vi "Out_S2F23.vi"(8 "error in (no error)":errorcluster, 10 "S2F23":T1, 11 "S2 Message Class in":refnum<class "S2 Message Class.lvclass">) -> (0 "error out":errorcluster, 3 "S2 Message Class out":refnum<class "S2 Message Class.lvclass">)   [LabVIEW 2020, in "SECS Communication.lvlib" / "S2 Message Class.lvclass"]
uses:
  S2 Message Class.lvclass
  D:/Dropbox/SECS/SECS_GEM v1.0.6/Com/SECS Communication/SECS-II Class/SECS-II Class.lvclass
  S2F23.ctl
  SECS-II Class/Data Message_List.vi
  SECS-II Class/Data Message_U4.vi
  SECS-II Class/Data Message_ASCII.vi
  SECS-II Class/SECS-II Class.lvclass
  D:/Dropbox/SECS/SECS_GEM v1.0.6/Com/SECS Communication/S2 Message Class/S2 Message Class.lvclass
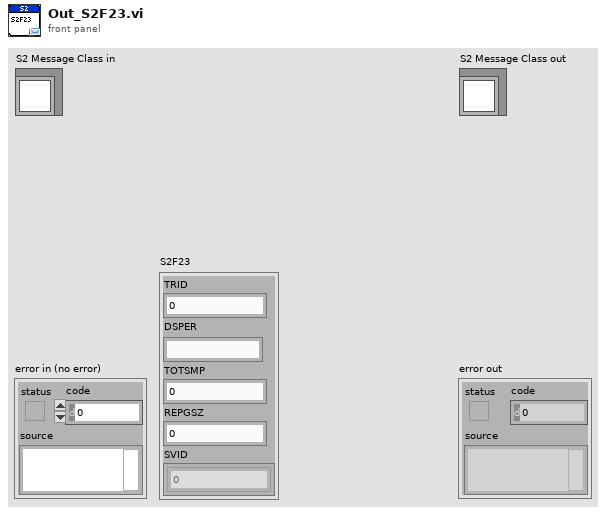
[diagram p1: front panel]
types:
  T1 = typedef "SECS Communication.lvlib/S2 Message Class.lvclass/S2F23.ctl" = cluster{"TRID":u32, "DSPER":string, "TOTSMP":u32, "REPGSZ":u32, "SVID":u32[]}
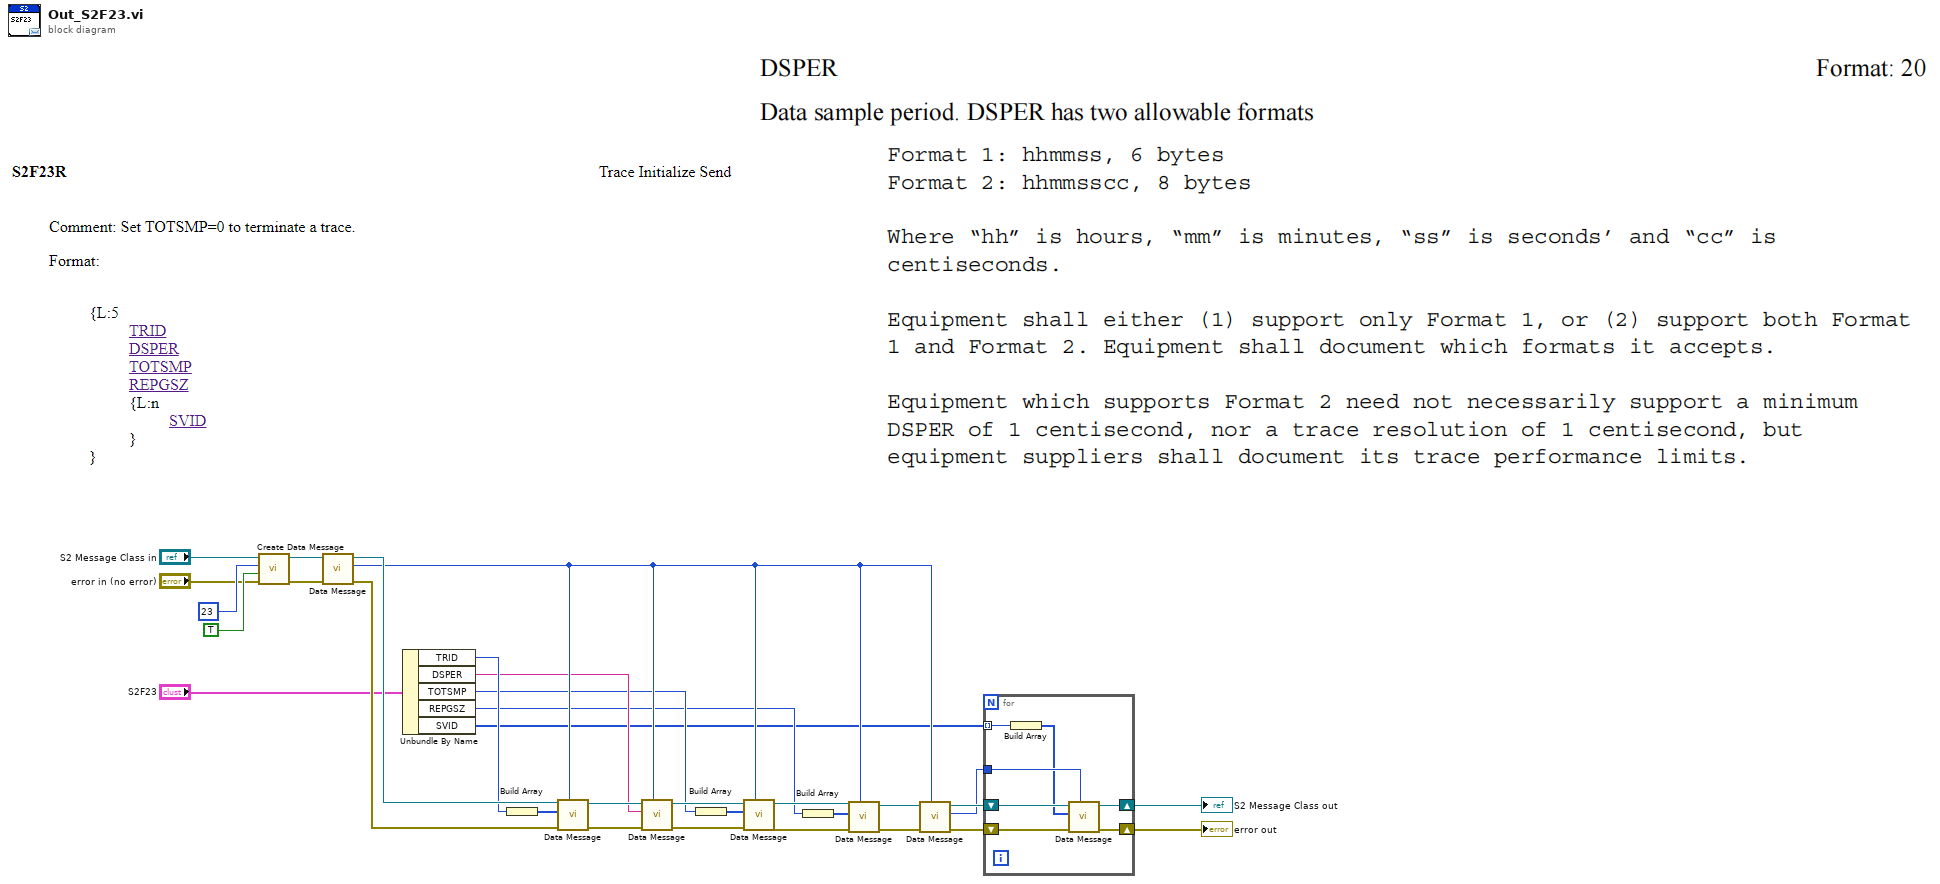
[diagram p0: block diagram]
diagram:
  n1 = call "Create Data Message.vi"("error in (no error)"="error in (no error)", "W-Bit"=TRUE, "Function"=u8 23, "SECS-II Class in"="S2 Message Class in") -> ("error out"=w28:errorcluster, "SECS-II Class out"=w29:refnum<class "S2 Message Class.lvclass">)  [unwired: 6 in]
  n2 = call-poly "Data Message.vi"("error in"=w28, "SECS-II Class in"=w29) -> ("error out"=w27:errorcluster, "Index"=w20:i32, "SECS-II Class out"=w26:refnum<class "S2 Message Class.lvclass">)  [unwired: 7 in]
  n3 = Unbundle By Name("S2F23") -> ("TRID"=w18:u32, "DSPER"=w15:string, "TOTSMP"=w11:u32, "REPGSZ"=w7:u32, "SVID"=w1:u32[])
  n4 = Build Array(w18) -> (w19:u32[])
  n5 = call-poly "Data Message.vi"("Parent Index"=w20, "error in"=w27, "Data"=w19, "SECS-II Class in"=w26) -> ("error out"=w16:errorcluster, "SECS-II Class out"=w17:refnum<class "S2 Message Class.lvclass">)  [unwired: 6 in]
  n6 = call-poly "Data Message.vi"("Parent Index"=w20, "error in"=w16, "Data"=w15, "SECS-II Class in"=w17) -> ("error out"=w13:errorcluster, "SECS-II Class out"=w14:refnum<class "S2 Message Class.lvclass">)  [unwired: 6 in]
  n7 = Build Array(w11) -> (w12:u32[])
  n8 = call-poly "Data Message.vi"("Parent Index"=w20, "error in"=w13, "Data"=w12, "SECS-II Class in"=w14) -> ("error out"=w8:errorcluster, "SECS-II Class out"=w9:refnum<class "S2 Message Class.lvclass">)  [unwired: 6 in]
  n9 = Build Array(w7) -> (w10:u32[])
  n10 = call-poly "Data Message.vi"("Parent Index"=w20, "error in"=w8, "Data"=w10, "SECS-II Class in"=w9) -> ("error out"=w5:errorcluster, "SECS-II Class out"=w6:refnum<class "S2 Message Class.lvclass">)  [unwired: 6 in]
  n11 = call-poly "Data Message.vi"("Parent Index"=w20, "error in"=w5, "SECS-II Class in"=w6) -> ("error out"=w3:errorcluster, "Index"=w2:i32, "SECS-II Class out"=w4:refnum<class "S2 Message Class.lvclass">)  [unwired: 6 in]
  n12 = for {
    shift-right: [w33] -> w23
    shift-left: w4 -> [w36]
    shift-right: [w32] -> w22
    shift-left: w3 -> [w37]
    tunnel: w2 -> [w35]
    tunnel: w1 -> [w38] mode=indexing
    n13 = Build Array(w38) -> (w34:u32[])
    n14 = call-poly "Data Message.vi"("Parent Index"=w35, "error in"=w37, "Data"=w34, "SECS-II Class in"=w36) -> ("error out"=w32:errorcluster, "SECS-II Class out"=w33:refnum<class "S2 Message Class.lvclass">)  [unwired: 6 in]
  }
  "error out" <- w22
  "S2 Message Class out" <- w23
